vi "LINX - SSD1306 OLED.vi"() -> ()   [LabVIEW 2011, in "LVH-LINX.lvlib"]
uses:
  vi.lib/LabVIEW Hacker/LINX/LVH-LINX.lvlib
  vi.lib/LabVIEW Hacker/LINX/Public/Sensors/Display/SSD1306/Private/SSD1306 Config.ctl
  vi.lib/LabVIEW Hacker/LINX/Public/Sensors/Display/SSD1306/SSD1306.lvlib
panel:
  out "Array":bool[][](array[boolean])
  in  "Image Path (128x32 PNG)":path
  in  "Stop Button":bool
  in  "SSD1306 Channels":T1={"SPI Channel (0)"=0, "VDD Channel"=38, "VBAT Channel"=40, "RESET Channel"=10, "DC Channel"=39, "SPI CS (3)"=0}
  in  "Serial Port":refnum<visa-resource-name>="COM3"
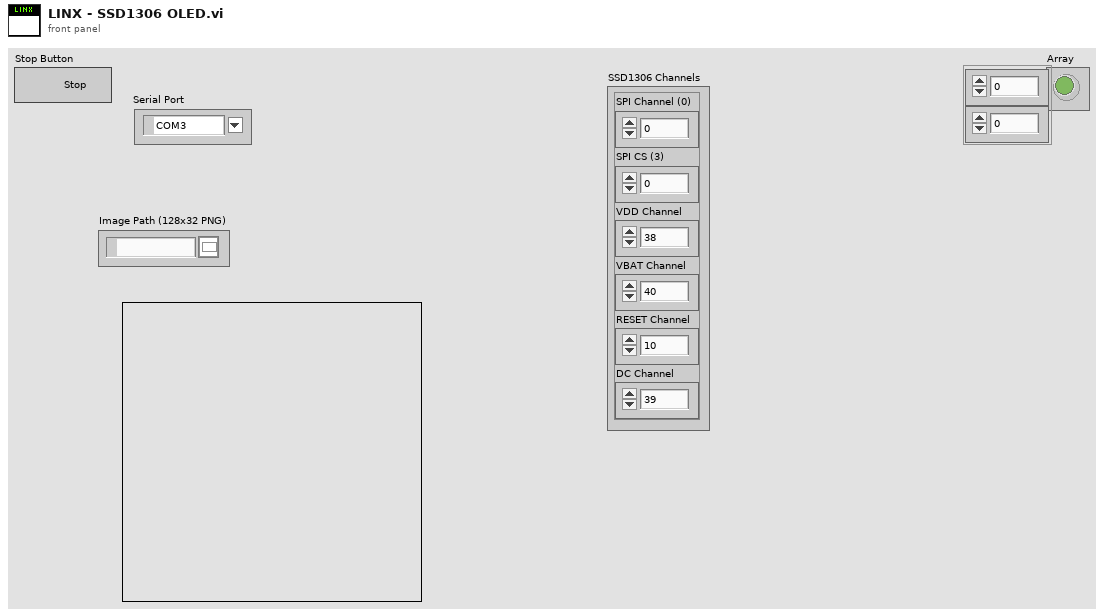
[diagram p1: front panel]
types:
  T1 = typedef "LVH-LINX.lvlib/SSD1306.lvlib/SSD1306 Config.ctl" = cluster{"SPI Channel (0)":u8, "VDD Channel":u8, "VBAT Channel":u8, "RESET Channel":u8, "DC Channel":u8, "SPI CS (3)":u8}
  T2 = typedef "LVH-LINX.lvlib/LINX Ref.ctl" = cluster{"Platform":T3, "Interface":T4, "LINX Device Config":T5}
  T3 = typedef "LVH-LINX.lvlib/Platform.ctl" = enum16{"LINX", "myRIO"}
  T4 = typedef "LVH-LINX.lvlib/Interface.ctl" = enum16{"Serial", "TCP"}
  T5 = typedef "LVH-LINX.lvlib/Device.lvlib/LINX Device Config.ctl" = cluster{"Interface":T4, "COM Port":refnum<visa-resource-name>, "TCP Configuration":T6, "Device Family":T7, "Device ID":u8, "Device Name":string, "TCP Ref":refnum<k5>}
  T6 = typedef "LVH-LINX.lvlib/Device.lvlib/TCP Config.ctl" = cluster{"IP Address":string, "Port":u16}
  T7 = typedef "LVH-LINX.lvlib/Device Family.ctl" = enum8{"National Instruments", "Digilent", "Arduino"}
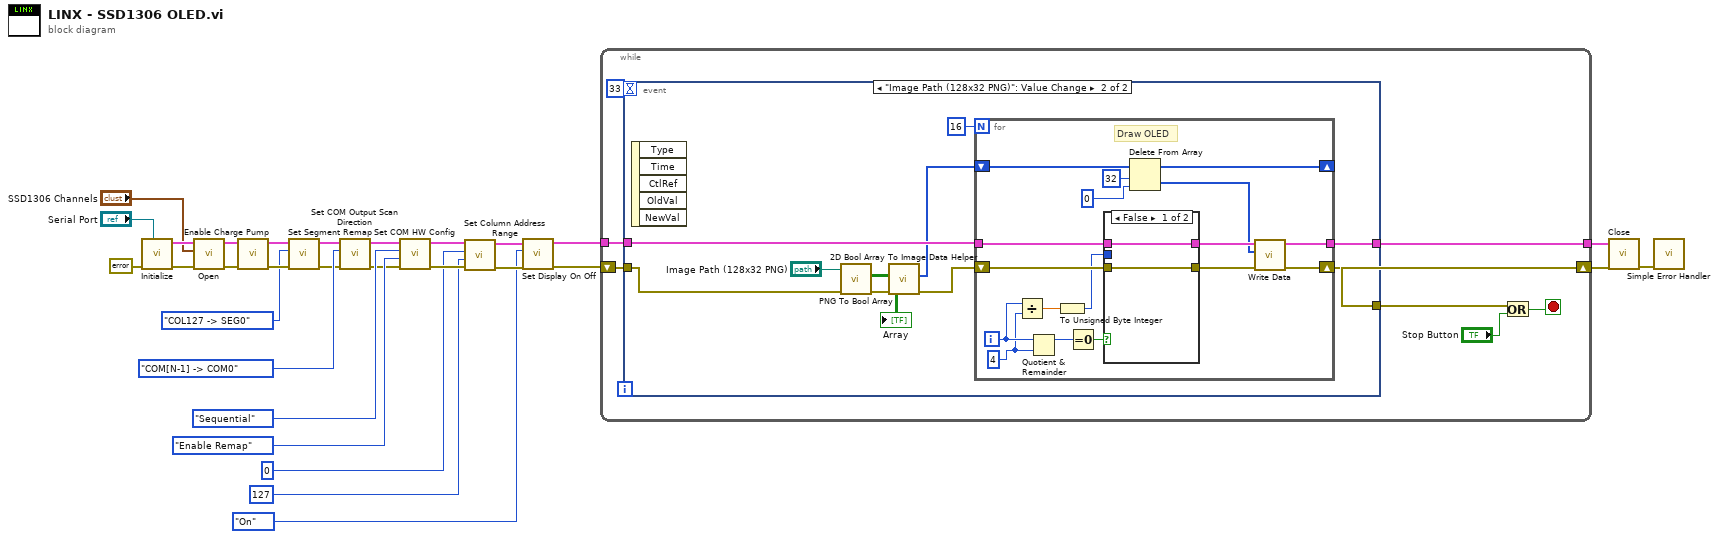
[diagram p0: block diagram]
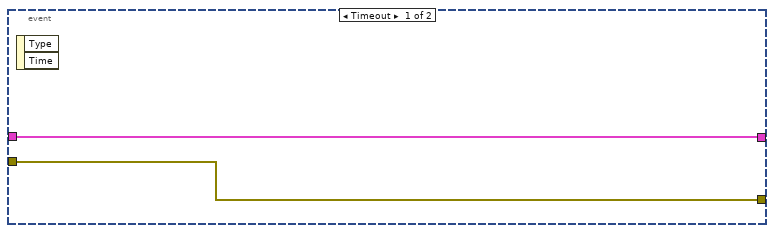
[diagram p2: hidden frame]
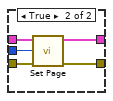
[diagram p3: hidden frame]
diagram:
  n1 = call "Initialize.vi"("Serial Port"="Serial Port", "Error In"=errorcluster {"status"=FALSE, "code"=0, "source"=""}) -> ("Error Out"=w25:errorcluster, "LINX Ref"=w26:T2)  [unwired: 7 in, 1 out]
  n2 = call "Open.vi"("Error In"=w25, "SSD1306 Channels"="SSD1306 Channels", "LINX Resource"=w26) -> ("Error Out"=w22:errorcluster, "LINX Resource"=w23:T2)  [unwired: 7 in]
  n3 = call "Enable Charge Pump.vi"("Error In"=w22, "LINX Resource"=w23) -> ("Error Out"=w21:errorcluster, "LINX Resource"=w20:T2)  [unwired: 8 in]
  n4 = call "Set Segment Remap.vi"("Error In"=w21, "Segment Remap"=enum8{"COL 0 -> SEG0", "COL127 -> SEG0"}."COL127 -> SEG0", "LINX Resource"=w20) -> ("Error Out"=w14:errorcluster, "LINX Resource"=w15:T2)  [unwired: 7 in]
  n5 = call "Set COM Output Scan Direction.vi"("Error In"=w14, "COM Direction"=enum8{"COM0 -> COM[N-1]", "COM[N-1] -> COM0"}."COM[N-1] -> COM0", "LINX Resource"=w15) -> ("Error Out"=w12:errorcluster, "LINX Resource"=w13:T2)  [unwired: 7 in]
  n6 = call "Set COM HW Config.vi"("Error In"=w12, "COM Left/Right Remap"=enum8{"Disable Remap", "Enable Remap"}."Enable Remap", "COM Pin Config"=enum8{"Sequential", "Alternative"}."Sequential", "LINX Resource"=w13) -> ("Error Out"=w11:errorcluster, "LINX Resource"=w10:T2)  [unwired: 6 in]
  n7 = call "Set Column Address Range.vi"("Error In"=w11, "Column End Address"=u8 127 ("Column Start Address"), "Column Start Address"=u8 0, "LINX Resource 2"=w10) -> ("Error Out"=w7:errorcluster, "LINX Resource"=w6:T2)  [unwired: 6 in]
  n8 = call "Set Display On Off.vi"("Error In"=w7, "Display On/Off"=enum8{"Off", "On"}."On", "LINX Resource 2"=w6) -> ("Error Out"=w4:errorcluster, "LINX Resource"=w3:T2)  [unwired: 7 in]
  n9 = while {
    tunnel: w3 -> [w34]
    shift-right: [w33] -> w2
    shift-left: w4 -> [w31]
    tunnel: [w32] -> w1
    stop <- w36 stop-if-true
    n10 = event shown="[1] \"Image Path (128x32 PNG)\": Value Change" {
      selector: _ -> [_ _]
      dyn-events: _ -> [_ _]
      timeout: 33 -> [_ _]
      tunnel: w34 -> [w37 w47]
      tunnel: [w38 w46] -> w33
      tunnel: [w37 w45] -> w32
      tunnel: w31 -> [w38 w42]
      event Timeout {
        n11 = event-data() -> ()  [unwired: 1 in, 2 out]
      }
      event "Image Path (128x32 PNG)": Value Change {
        n12 = event-data() -> ()  [unwired: 1 in, 5 out]
        n13 = call "PNG To Bool Array.vi"("Error In"=w42, "path to PNG file"="Image Path (128x32 PNG)") -> ("Error Out"=w44:errorcluster, "Array"=w41:bool[][])  [unwired: 8 in]
        "Array" <- w41
        n14 = call "2D Bool Array To Image Data Helper.vi"("Error In"=w44, "Image Data"=w41) -> ("Error Out"=w43:errorcluster, "Image Data"=w40:u8[])  [unwired: 8 in]
        n15 = for {
          N: 16 -> [_]
          tunnel: w47 -> [w58]
          shift-right: [w54] -> _
          shift-left: w40 -> [w55]
          shift-right: [w50] -> w46
          shift-left: w43 -> [w63]
          tunnel: [w49] -> w45
          i -> [w62]
          w61 = 4 ("y")
          # "Draw OLED"
          n16 = Divide(x=w62, y=w61) -> (x/y=w60:dbl)
          n17 = Quotient & Remainder(x=w62, y=w61) -> (x-y*floor(x/y)=w65:i32)  [unwired: 1 out]
          n18 = To Unsigned Byte Integer(number=w60) -> (unsigned 8bit integer=w59:u8)
          n19 = Equal To 0?(x=w65) -> (x = 0?=w64:bool)
          n20 = case shown="False" w64 {
            tunnel: w63 -> [w66 w72]
            tunnel: w59 -> [_ w71]
            tunnel: w58 -> [w67 w70]
            tunnel: [w66 w69] -> w57
            tunnel: [w67 w68] -> w56
            frame False {
            }
            frame True {
              n21 = call "Set Page.vi"("Error In"=w72, "Page Address"=w71, "LINX Resource"=w70) -> ("Error Out"=w69:errorcluster, "LINX Resource"=w68:T2)  [unwired: 7 in]
            }
          }
          n22 = Delete From Array(array=w55, length=32, index=0) -> (deleted portion=w51:u8[], array with subset deleted=w54:u8[])
          n23 = call "Write Data.vi"("Error In"=w57, "Data"=w51, "LINX Resource"=w56) -> ("Error Out"=w50:errorcluster, "LINX Resource"=w49:T2)  [unwired: 7 in]
        }
      }
    }
    n24 = Or(x=w33, y="Stop Button") -> (x .or. y?=w36:bool)
  }
  n25 = call "Close.vi"("Error In"=w2, "LINX Resource"=w1) -> ("Error Out"=w28:errorcluster)  [unwired: 8 in, 1 out]
  n26 = call <vilib>:"Simple Error Handler.vi"("error in (no error)"=w28) -> ()  [unwired: 4 in, 5 out]
